vi "List Basic Types.vi"() -> (1 "Short Class Names":string[](array[string]), 2 "Long Class Names":string[](array[string]), 3 "Basic Types":refnum<class "Tree Data.lvclass">[](array[class]))   [LabVIEW 2020, in "NI_VIAnCFGDataStructure.lvlib" / "Tree.lvclass"]
doc: "Return a list of all basic Tree Data types used by Tree API"
uses:
  <vilib>/addons/analyzer/VIAnCFGDataStructure/Tree Manager/Tree.lvclass
  <vilib>/addons/analyzer/VIAnCFGDataStructure/Tree Data/Tree Data.lvclass
  <vilib>/addons/analyzer/VIAnCFGDataStructure/Data Types/2D String/2D String.lvclass
  e:/builds/penguin/labview/branches/2020/dev/dist/vi.lib/addons/analyzer/VIAnCFGDataStructure/Tree Data/Tree Data.lvclass
  <vilib>/addons/analyzer/VIAnCFGDataStructure/Data Types/2D Path/2D Path.lvclass
  <vilib>/addons/analyzer/VIAnCFGDataStructure/Data Types/2D Flt/2D Flt.lvclass
  <vilib>/addons/analyzer/VIAnCFGDataStructure/Data Types/2D Int/2D Int.lvclass
  <vilib>/addons/analyzer/VIAnCFGDataStructure/Data Types/2D Bool/2D Bool.lvclass
  <vilib>/addons/analyzer/VIAnCFGDataStructure/Data Types/String/String.lvclass
  <vilib>/addons/analyzer/VIAnCFGDataStructure/Data Types/String Array/1D String.lvclass
  <vilib>/addons/analyzer/VIAnCFGDataStructure/Data Types/Path/Path.lvclass
  <vilib>/addons/analyzer/VIAnCFGDataStructure/Data Types/Path Array/1D Path.lvclass
  <vilib>/addons/analyzer/VIAnCFGDataStructure/Data Types/Int/Int.lvclass
  <vilib>/addons/analyzer/VIAnCFGDataStructure/Data Types/Int Array/1D Int.lvclass
  <vilib>/addons/analyzer/VIAnCFGDataStructure/Data Types/Float/Flt.lvclass
  <vilib>/addons/analyzer/VIAnCFGDataStructure/Data Types/Flt Array/1D Flt.lvclass
  <vilib>/addons/analyzer/VIAnCFGDataStructure/Data Types/Bool/Bool.lvclass
  <vilib>/addons/analyzer/VIAnCFGDataStructure/Data Types/Bool Array/1D Bool.lvclass
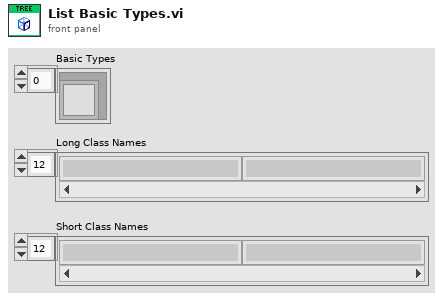
[diagram p1: front panel]
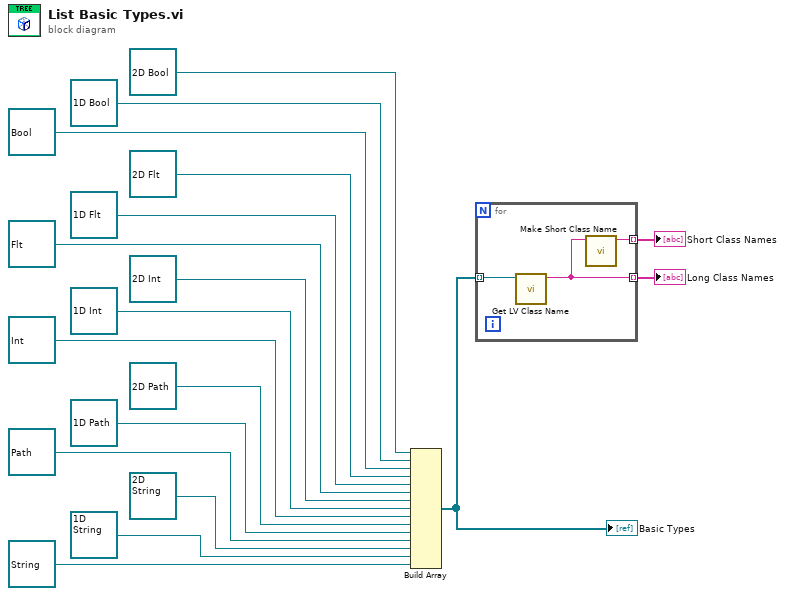
[diagram p0: block diagram]
diagram:
  n1 = Build Array(refnum<class "2D Bool.lvclass"> refnum ("Tree API.lvlib:2D Bool.lvclass"), refnum<class "1D Bool.lvclass"> refnum ("Bool Array.lvclass"), refnum<class "Bool.lvclass"> refnum ("Bool.lvclass"), refnum<class "2D Flt.lvclass"> refnum ("Tree API.lvlib:2D Flt.lvclass"), refnum<class "1D Flt.lvclass"> refnum ("Flt Array.lvclass"), refnum<class "Flt.lvclass"> refnum ("Flt.lvclass"), refnum<class "2D Int.lvclass"> refnum ("Tree API.lvlib:2D Int.lvclass"), refnum<class "1D Int.lvclass"> refnum ("Int Array.lvclass"), refnum<class "Int.lvclass"> refnum ("Int.lvclass"), refnum<class "2D Path.lvclass"> refnum ("Tree API.lvlib:2D Path.lvclass"), refnum<class "1D Path.lvclass"> refnum ("Path Array.lvclass"), refnum<class "Path.lvclass"> refnum ("Path.lvclass"), refnum<class "2D String.lvclass"> refnum ("Tree API.lvlib:2D String.lvclass"), refnum<class "1D String.lvclass"> refnum ("String Array.lvclass"), refnum<class "String.lvclass"> refnum ("String.lvclass")) -> (w7:refnum<class "Tree Data.lvclass">[])
  "Basic Types" <- w7
  n2 = for {
    tunnel: w7 -> [w21] mode=indexing
    tunnel: [w20] -> w8 mode=indexing
    tunnel: [w19] -> w6 mode=indexing
    n3 = call <vilib>:"Get LV Class Name.vi"("object"=w21) -> ("class name"=w20:string)  [unwired: 9 in, 1 out]
    n4 = call <vilib>:"Make Short Class Name.vi"("Class Name"=w20) -> ("Shortened Class Name"=w19:string)  [unwired: 10 in]
  }
  "Long Class Names" <- w8
  "Short Class Names" <- w6
